vi "List Tags By Type.vi"(8 "error in (no error)":errorcluster, 9 "NI Specific Type":T2, 10 "Broad Types":T1, 11 "Var Bus in":refnum<class "Var Bus.lvclass">) -> (0 "error out":errorcluster, 2 "Tags":string[](array[string]), 3 "Var Bus out":refnum<class "Var Bus.lvclass">)   [LabVIEW 2021, in "Var Bus.lvclass"]
uses:
  Var Bus.lvclass
  <vilib>/Utility/Data Type/Type Definitions/Data Type.ctl
  Support/Broad Types.ctl
  Var Bus.lvclass/Var Bus.ctl
  LV_Abstract/Source/Abs_Types/Value/Abs_Value.lvclass
  LV_Abstract/Source/Abs_Types/Numeric/Abs_Numeric.lvclass
  LV_Abstract/Source/Abs_Types/Floating Point/Abs_Floating Point.lvclass
  LV_Abstract/Source/Abs_Types/Boolean/Abs_Boolean.lvclass
  LV_Abstract/Source/Abs_Types/String/Abs_String.lvclass
  LV_Abstract/Source/Abs_Types/Integer/Abs_Integer.lvclass
  Properties/Read Var Map.vi
  LV_Abstract/Source/Abs_Types/Type/Abs_Type.lvclass
  <vilib>/Utility/Data Type/NI_Data Type.lvlib
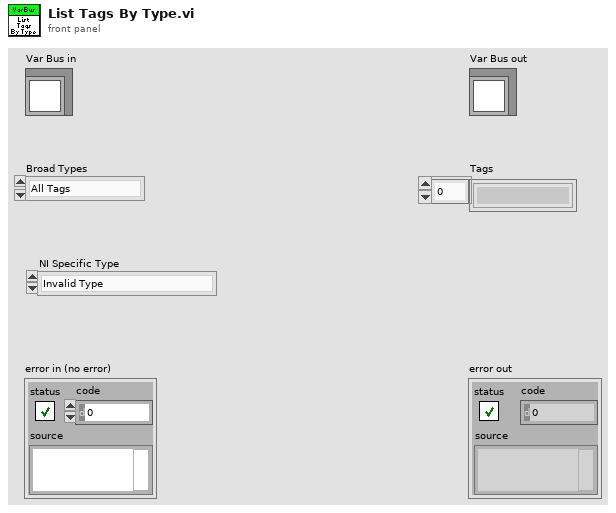
[diagram p1: front panel]
types:
  T1 = typedef "Var Bus.lvclass/Broad Types.ctl" = enum16{"All Tags", "NI Specific Type", "Boolean", "String", "Numeric", "Float", "Integer", "Collection"}
  T2 = typedef "NI_Data Type.lvlib/Data Type.ctl" = enum8{"Invalid Type", "Void", "I8", "I16", "I32", "I64", "U8", "U16", "U32", "U64", "Single Float", "Double Float", "Extended Float", "Single Complex", "Double Complex", "Extended Complex", "Enum U8", "Enum U16", "Enum U32", "Enum U64", "Single Float With Unit", "Double Float With Unit", "Extended Float With Unit", "Single Complex with Unit", "Double Complex with Unit", "Extended Complex with Unit", "Boolean", "String", "Path", "Picture", "Tag", "Array", "Cluster", "Variant", "LV Variant", "Waveform", "Timestamp", "Digital Waveform", "Digital Data", "ExpressData", "Refnum", "External Data", "VI", "Poly VI", "LabVIEW Class Instance", "Fixed Point", "Set Collection", "Map Collection"}
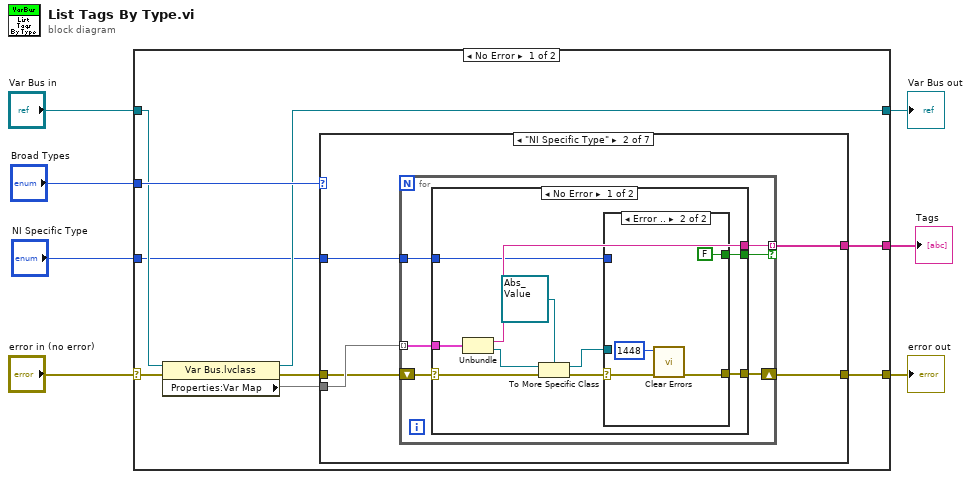
[diagram p0: block diagram]
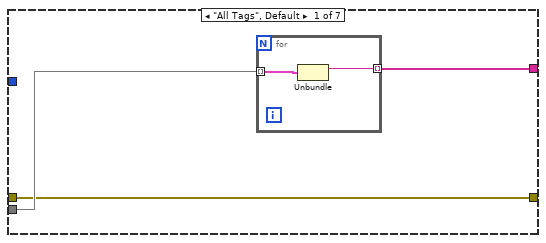
[diagram p2: hidden frame]
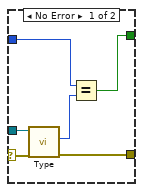
[diagram p3: hidden frame]
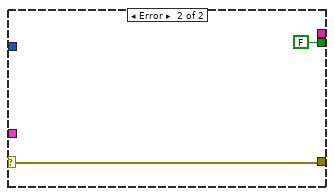
[diagram p4: hidden frame]
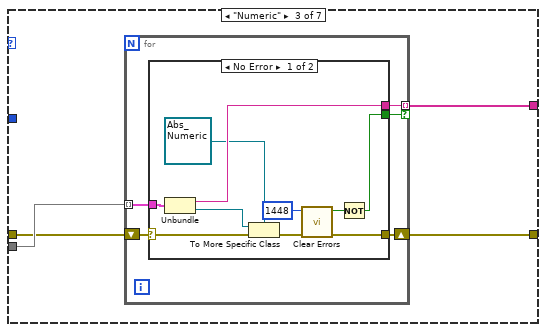
[diagram p5: hidden frame]
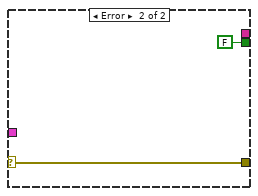
[diagram p6: hidden frame]
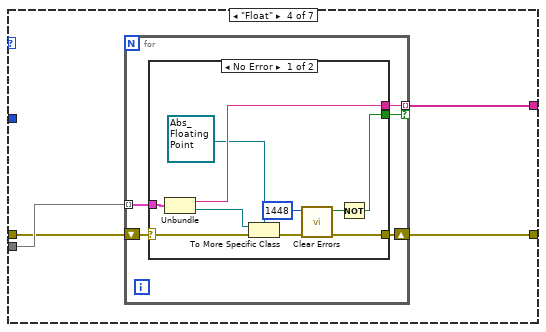
[diagram p7: hidden frame]
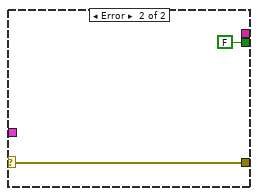
[diagram p8: hidden frame]
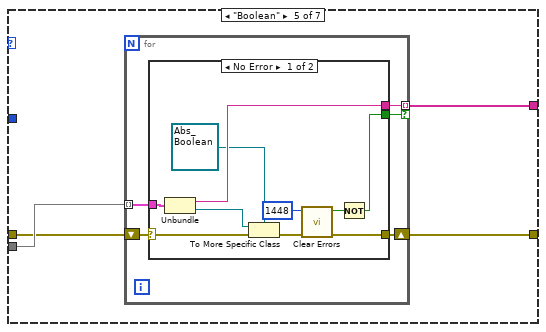
[diagram p9: hidden frame]
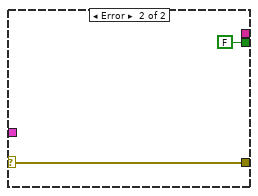
[diagram p10: hidden frame]
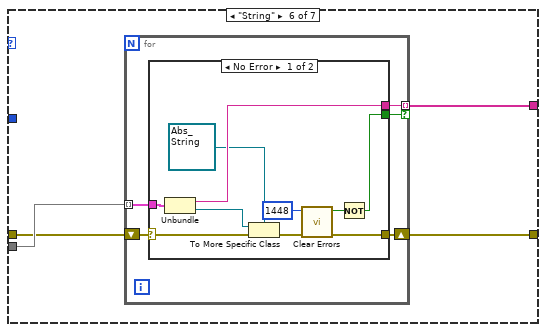
[diagram p11: hidden frame]
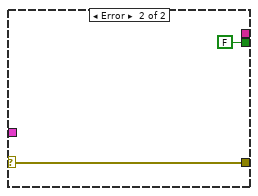
[diagram p12: hidden frame]
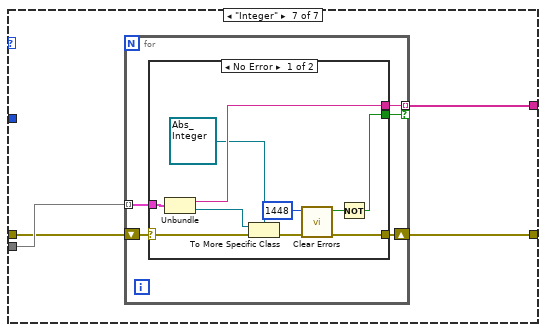
[diagram p13: hidden frame]
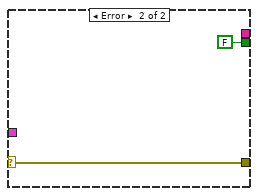
[diagram p14: hidden frame]
diagram:
  n1 = case shown="No Error" "error in (no error)" {
    selector: "error in (no error)" -> [w10 w161]
    tunnel: [w9 w161] -> w6
    tunnel: [w13 w160] -> w4
    tunnel: "Var Bus in" -> [w14 w160]
    tunnel: "Broad Types" -> [w16 _]
    tunnel: [w15 _] -> w2
    tunnel: "NI Specific Type" -> [w8 _]
    frame No Error {
      n2 = property class="Var Bus.lvclass"(reference=w14, error in=w10) -> (reference out=w13:refnum<class "Var Bus.lvclass">, error out=w11:errorcluster, "Properties:Var Map"=w12:map{string, refnum<class "Abs_Type.lvclass">})
      n3 = case shown="\"NI Specific Type\"" w16 {
        tunnel: w11 -> [w17 w24 w56 w77 w98 w119 w140]
        tunnel: [w17 w22 w55 w76 w97 w118 w139] -> w9
        tunnel: [w19 w26 w58 w79 w100 w121 w142] -> w15
        tunnel: w12 -> [w18 w25 w57 w78 w99 w120 w141]
        tunnel: w8 -> [_ w23 _ _ _ _ _]
        frame "All Tags", Default {
          n4 = for {
            tunnel: w18 -> [w21] mode=indexing
            tunnel: [w20] -> w19 mode=indexing
            n5 = Unbundle(w21) -> (w20:string)  [unwired: 1 out]
          }
        }
        frame "NI Specific Type" {
          n6 = for {
            tunnel: w25 -> [w32] mode=indexing
            tunnel: [w31] -> w26 mode=indexing if=w28
            shift-right: [w30] -> w22
            shift-left: w24 -> [w27]
            tunnel: w23 -> [w29]
            n7 = case shown="No Error" w27 {
              selector: w27 -> [w37 w53]
              tunnel: w32 -> [w42 _]
              tunnel: [w41 _] -> w31
              tunnel: [w40 w53] -> w30
              tunnel: w29 -> [w39 _]
              tunnel: [w38 FALSE] -> w28
              frame No Error {
                n8 = Unbundle(w42) -> (w41:string, "Abs_Type.lvclass"=w35:refnum<class "Abs_Type.lvclass">)
                n9 = To More Specific Class(target class=refnum<class "Abs_Value.lvclass"> refnum ("Abs_Value.lvclass"), reference=w35, error in=w37) -> (specific class reference=w33:refnum<class "Abs_Value.lvclass">, error out=w36:errorcluster)
                n10 = case shown="Error .." w36 {
                  selector: w36 -> [w44 w52]
                  tunnel: [w48 w51] -> w40
                  tunnel: w39 -> [w46 _]
                  tunnel: [w45 FALSE] -> w38
                  tunnel: w33 -> [w43 _]
                  frame No Error {
                    n11 = call-dynamic "Type.vi"("error in (no error)"=w44, "Element in"=w43) -> ("error out"=w48:errorcluster, "Type"=w47:T2)  [unwired: 7 in, 1 out]
                    n12 = Equal?(x=w46, y=w47) -> (x = y?=w45:bool)
                  }
                  frame Error {
                    n13 = call <vilib>:"Clear Errors.vi"("error in (no error)"=w52, "specific error code to clear (0: all)"=1448) -> ("error out"=w51:errorcluster)  [unwired: 4 in, 1 out]
                  }
                }
              }
              frame Error {
              }
            }
          }
        }
        frame "Numeric" {
          n14 = for {
            tunnel: w57 -> [w63] mode=indexing
            tunnel: [w62] -> w58 mode=indexing if=w59
            shift-right: [w60] -> w55
            shift-left: w56 -> [w61]
            n15 = case shown="No Error" w61 {
              selector: w61 -> [w71 w75]
              tunnel: w63 -> [w73 _]
              tunnel: [w72 _] -> w62
              tunnel: [w67 w75] -> w60
              tunnel: [w65 FALSE] -> w59
              frame No Error {
                n16 = Unbundle(w73) -> (w72:string, "Abs_Type.lvclass"=w69:refnum<class "Abs_Type.lvclass">)
                n17 = To More Specific Class(target class=refnum<class "Abs_Numeric.lvclass"> refnum ("Abs_Numeric.lvclass"), reference=w69, error in=w71) -> (error out=w68:errorcluster)  [unwired: 1 out]
                n18 = call <vilib>:"Clear Errors.vi"("error in (no error)"=w68, "specific error code to clear (0: all)"=1448) -> ("error out"=w67:errorcluster, "specific error cleared?"=w66:bool)  [unwired: 4 in]
                n19 = Not(x=w66) -> (.not. x?=w65:bool)
              }
              frame Error {
              }
            }
          }
        }
        frame "Float" {
          n20 = for {
            tunnel: w78 -> [w84] mode=indexing
            tunnel: [w83] -> w79 mode=indexing if=w80
            shift-right: [w81] -> w76
            shift-left: w77 -> [w82]
            n21 = case shown="No Error" w82 {
              selector: w82 -> [w92 w96]
              tunnel: w84 -> [w94 _]
              tunnel: [w93 _] -> w83
              tunnel: [w89 w96] -> w81
              tunnel: [w87 FALSE] -> w80
              frame No Error {
                n22 = Unbundle(w94) -> (w93:string, "Abs_Type.lvclass"=w91:refnum<class "Abs_Type.lvclass">)
                n23 = To More Specific Class(target class=refnum<class "Abs_Floating Point.lvclass"> refnum ("Abs_Floating Point.lvclass"), reference=w91, error in=w92) -> (error out=w90:errorcluster)  [unwired: 1 out]
                n24 = call <vilib>:"Clear Errors.vi"("error in (no error)"=w90, "specific error code to clear (0: all)"=1448) -> ("error out"=w89:errorcluster, "specific error cleared?"=w88:bool)  [unwired: 4 in]
                n25 = Not(x=w88) -> (.not. x?=w87:bool)
              }
              frame Error {
              }
            }
          }
        }
        frame "Boolean" {
          n26 = for {
            tunnel: w99 -> [w105] mode=indexing
            tunnel: [w104] -> w100 mode=indexing if=w101
            shift-right: [w102] -> w97
            shift-left: w98 -> [w103]
            n27 = case shown="No Error" w103 {
              selector: w103 -> [w113 w117]
              tunnel: w105 -> [w115 _]
              tunnel: [w114 _] -> w104
              tunnel: [w110 w117] -> w102
              tunnel: [w108 FALSE] -> w101
              frame No Error {
                n28 = Unbundle(w115) -> (w114:string, "Abs_Type.lvclass"=w112:refnum<class "Abs_Type.lvclass">)
                n29 = To More Specific Class(target class=refnum<class "Abs_Boolean.lvclass"> refnum ("Abs_Boolean.lvclass"), reference=w112, error in=w113) -> (error out=w111:errorcluster)  [unwired: 1 out]
                n30 = call <vilib>:"Clear Errors.vi"("error in (no error)"=w111, "specific error code to clear (0: all)"=1448) -> ("error out"=w110:errorcluster, "specific error cleared?"=w109:bool)  [unwired: 4 in]
                n31 = Not(x=w109) -> (.not. x?=w108:bool)
              }
              frame Error {
              }
            }
          }
        }
        frame "String" {
          n32 = for {
            tunnel: w120 -> [w126] mode=indexing
            tunnel: [w125] -> w121 mode=indexing if=w122
            shift-right: [w123] -> w118
            shift-left: w119 -> [w124]
            n33 = case shown="No Error" w124 {
              selector: w124 -> [w134 w138]
              tunnel: w126 -> [w136 _]
              tunnel: [w135 _] -> w125
              tunnel: [w131 w138] -> w123
              tunnel: [w129 FALSE] -> w122
              frame No Error {
                n34 = Unbundle(w136) -> (w135:string, "Abs_Type.lvclass"=w133:refnum<class "Abs_Type.lvclass">)
                n35 = To More Specific Class(target class=refnum<class "Abs_String.lvclass"> refnum ("Abs_String.lvclass"), reference=w133, error in=w134) -> (error out=w132:errorcluster)  [unwired: 1 out]
                n36 = call <vilib>:"Clear Errors.vi"("error in (no error)"=w132, "specific error code to clear (0: all)"=1448) -> ("error out"=w131:errorcluster, "specific error cleared?"=w130:bool)  [unwired: 4 in]
                n37 = Not(x=w130) -> (.not. x?=w129:bool)
              }
              frame Error {
              }
            }
          }
        }
        frame "Integer" {
          n38 = for {
            tunnel: w141 -> [w147] mode=indexing
            tunnel: [w146] -> w142 mode=indexing if=w143
            shift-right: [w144] -> w139
            shift-left: w140 -> [w145]
            n39 = case shown="No Error" w145 {
              selector: w145 -> [w155 w159]
              tunnel: w147 -> [w157 _]
              tunnel: [w156 _] -> w146
              tunnel: [w152 w159] -> w144
              tunnel: [w150 FALSE] -> w143
              frame No Error {
                n40 = Unbundle(w157) -> (w156:string, "Abs_Type.lvclass"=w154:refnum<class "Abs_Type.lvclass">)
                n41 = To More Specific Class(target class=refnum<class "Abs_Integer.lvclass"> refnum ("Abs_Integer.lvclass"), reference=w154, error in=w155) -> (error out=w153:errorcluster)  [unwired: 1 out]
                n42 = call <vilib>:"Clear Errors.vi"("error in (no error)"=w153, "specific error code to clear (0: all)"=1448) -> ("error out"=w152:errorcluster, "specific error cleared?"=w151:bool)  [unwired: 4 in]
                n43 = Not(x=w151) -> (.not. x?=w150:bool)
              }
              frame Error {
              }
            }
          }
        }
      }
    }
    frame Error {
    }
  }
  "error out" <- w6
  "Var Bus out" <- w4
  "Tags" <- w2
